vi "Move To Name.vi"(4 "Return to Current":bool=TRUE, 5 "Motion Order":T1(ring)=enum."Auto", 6 "Direct":bool, 7 "Move if Same":bool=TRUE, 8 "error in":errorcluster, 9 "Speed(mm/s)":dbl=-1.0, 10 "Destination":string, 11 "Gantry in":refnum<class "Gantry.lvclass">) -> (0 "error out":errorcluster, 1 "Point Names":string[](array[string]), 3 "Gantry out":refnum<class "Gantry.lvclass">)   [LabVIEW 2024, in "Gantry.lvclass"]
uses:
  Gantry.lvclass
  Gantry.lvclass/Gantry.ctl
  FlexWorktable/FlexWorktable.lvclass
  Vec3d Class/Vec3d.lvclass
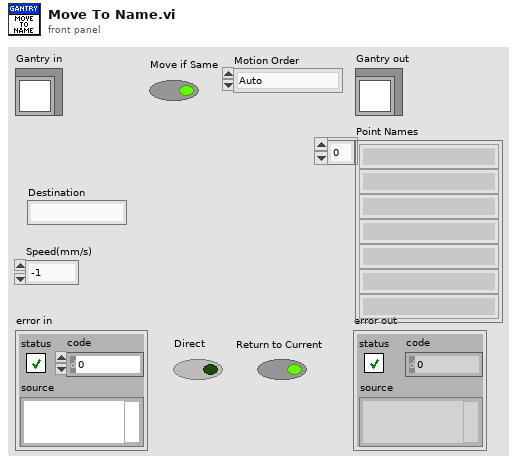
[diagram p1: front panel]
types:
  T1 = enum16{"Vertical First", "Lateral First", "Auto"}
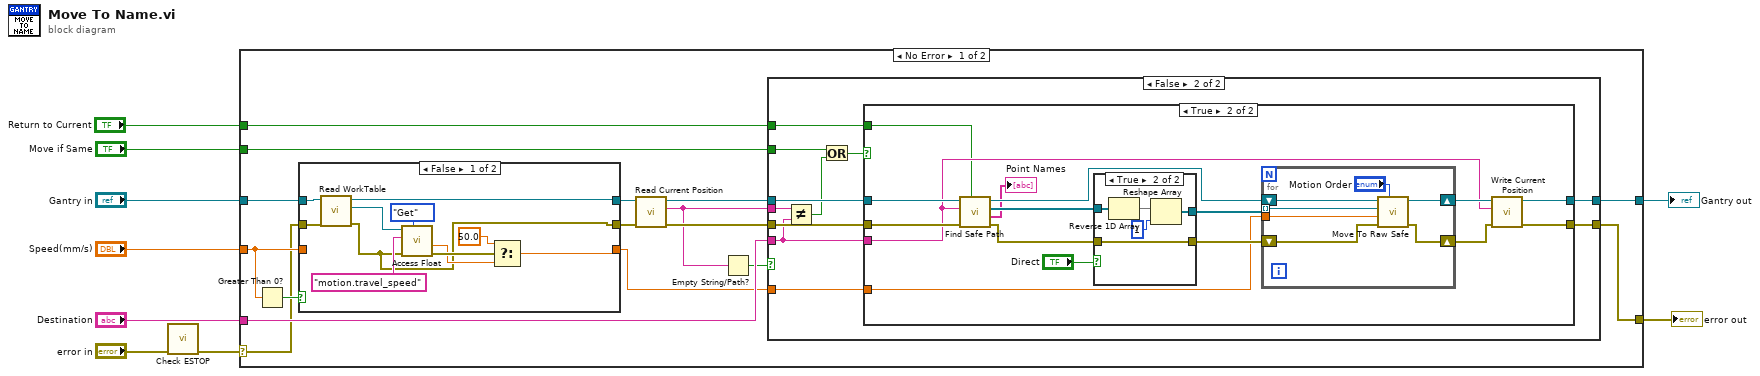
[diagram p0: block diagram]
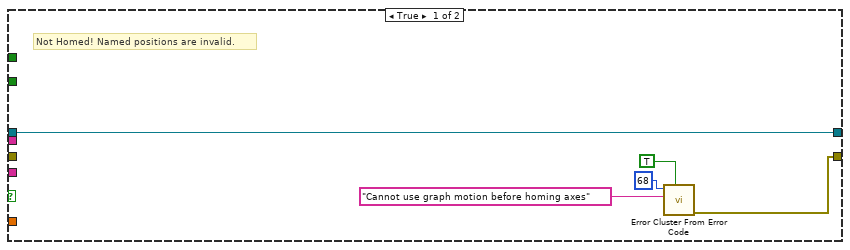
[diagram p3: hidden frame]
diagram:
  n1 = call "Check ESTOP.vi"("error in"="error in") -> ("error out"=w4:errorcluster)  [unwired: 10 in]
  n2 = case shown="No Error" w4 {
    selector: w4 -> [w14 w88]
    tunnel: [w25 w89] -> w9
    tunnel: "Gantry in" -> [w13 w89]
    tunnel: "Destination" -> [w21 _]
    tunnel: [w24 w88] -> w8
    tunnel: "Move if Same" -> [w20 _]
    tunnel: "Speed(mm/s)" -> [w16 _]
    tunnel: "Return to Current" -> [w10 _]
    frame No Error {
      n3 = Greater Than 0?(x=w16) -> (x > 0?=w17:bool)
      n4 = case shown="False" w17 {
        tunnel: w16 -> [_ w39]
        tunnel: [w27 w39] -> w15
        tunnel: w14 -> [w35 w37]
        tunnel: w13 -> [w36 w38]
        tunnel: [w34 w38] -> w12
        tunnel: [w26 w37] -> w11
        frame False {
          n5 = call-dynamic "Read WorkTable.vi"("error in"=w35, "Gantry Class in"=w36) -> ("error out"=w26:errorcluster, "Worktable"=w33:refnum<class "FlexWorktable.lvclass">, "Gantry Class out"=w34:refnum<class "Gantry.lvclass">)  [unwired: 7 in]
          n6 = call-dynamic "Access Float.vi"("Get/Set"=enum16{"Get", "Set"}."Get", "error in (no error)"=w26, "Key"="motion.travel_speed", "FlexWorktable in"=w33) -> ("error out"=w30:errorcluster, "Value out"=w28:dbl)  [unwired: 5 in, 1 out]
          n7 = Select(t=50.0, s=w30, f=w28) -> (s? t:f=w27:dbl)
        }
        frame True {
        }
      }
      n8 = call-dynamic "Read Current Position.vi"("error in"=w11, "Gantry in"=w12) -> ("error out"=w23:errorcluster, "Current Position"=w18:string, "Gantry out"=w22:refnum<class "Gantry.lvclass">)  [unwired: 7 in]
      n9 = Empty String/Path?(string/path=w18) -> (empty?=w19:bool)
      n10 = case shown="False" w19 {
        tunnel: [w44 w55] -> w25
        tunnel: [w43 w54] -> w24
        tunnel: w23 -> [_ w53]
        tunnel: w22 -> [w44 w52]
        tunnel: w18 -> [_ w51]
        tunnel: w21 -> [_ w50]
        tunnel: w20 -> [_ w49]
        tunnel: w15 -> [_ w46]
        tunnel: w10 -> [_ w45]
        frame True {
          # "Not Homed! Named positions are invalid."
          n11 = call <vilib>:"Error Cluster From Error Code.vi"("show call chain? (False)"=TRUE, "error message (\"\")"="Cannot use graph motion before homing axes", "error code (0)"=68) -> ("error out"=w43:errorcluster)  [unwired: 6 in]
        }
        frame False {
          n12 = Not Equal?(x=w51, y=w50) -> (x != y?=w47:bool)
          n13 = Or(x=w49, y=w47) -> (x .or. y?=w48:bool)
          n14 = case shown="True" w48 {
            tunnel: [w57 w73] -> w55
            tunnel: [w56 w70] -> w54
            tunnel: w46 -> [_ w61]
            tunnel: w53 -> [w56 w62]
            tunnel: w52 -> [w57 w63]
            tunnel: w50 -> [_ w60]
            tunnel: w45 -> [_ w59]
            frame False {
            }
            frame True {
              n15 = call-dynamic "Find Safe Path.vi"("Include Start"=w59, "error in"=w62, "Destination"=w60, "Gantry in"=w63) -> ("error out"=w64:errorcluster, "Point Names"=→"Point Names":string[], "Points Array"=w68:refnum<class "Vec3d.lvclass">[], "Gantry out"=w69:refnum<class "Gantry.lvclass">)  [unwired: 3 in]
              n16 = case shown="True" "Direct" {
                tunnel: w68 -> [w75 w80]
                tunnel: [w75 w78] -> w66
                tunnel: [w74 w76] -> w65
                tunnel: w64 -> [w74 w76]
                frame False {
                }
                frame True {
                  n17 = Reverse 1D Array(array=w80) -> (reversed array=w79:refnum<class "Vec3d.lvclass">[])
                  n18 = Reshape Array(w79, 1 ("dimension size")) -> (w78:refnum<class "Vec3d.lvclass">[])
                }
              }
              n19 = for {
                tunnel: w66 -> [w86] mode=indexing
                tunnel: w61 -> [w85]
                shift-right: [w83] -> w72
                shift-left: w69 -> [w87]
                shift-right: [w82] -> w71
                shift-left: w65 -> [w84]
                n20 = call-dynamic "Move To Raw Safe.vi"("Motion Order"="Motion Order", "error in"=w84, "Speed(mm/s)"=w85, "Destination"=w86, "Gantry in"=w87) -> ("error out"=w82:errorcluster, "Gantry out"=w83:refnum<class "Gantry.lvclass">)  [unwired: 5 in]
              }
              n21 = call-dynamic "Write Current Position.vi"("error in"=w71, "Current Position"=w60, "Gantry in"=w72) -> ("error out"=w70:errorcluster, "Gantry out"=w73:refnum<class "Gantry.lvclass">)  [unwired: 7 in]
            }
          }
        }
      }
    }
    frame Error {
    }
  }
  "error out" <- w8
  "Gantry out" <- w9
